vi "VCM_set_values.vi"(4 "Steps":i32=50, 5 "Frequenz":dbl, 6 "A max":dbl, 7 "Amplitude SET":dbl, 8 "mode":u16(ring), 9 "delay time":dbl, 10 "address":string) -> (2 "iter":i32, 3 "Amplitude IST":dbl)   [LabVIEW 2019]
panel:
  out "F-format string":string
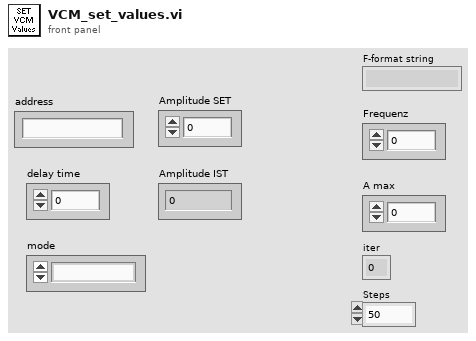
[diagram p1: front panel]
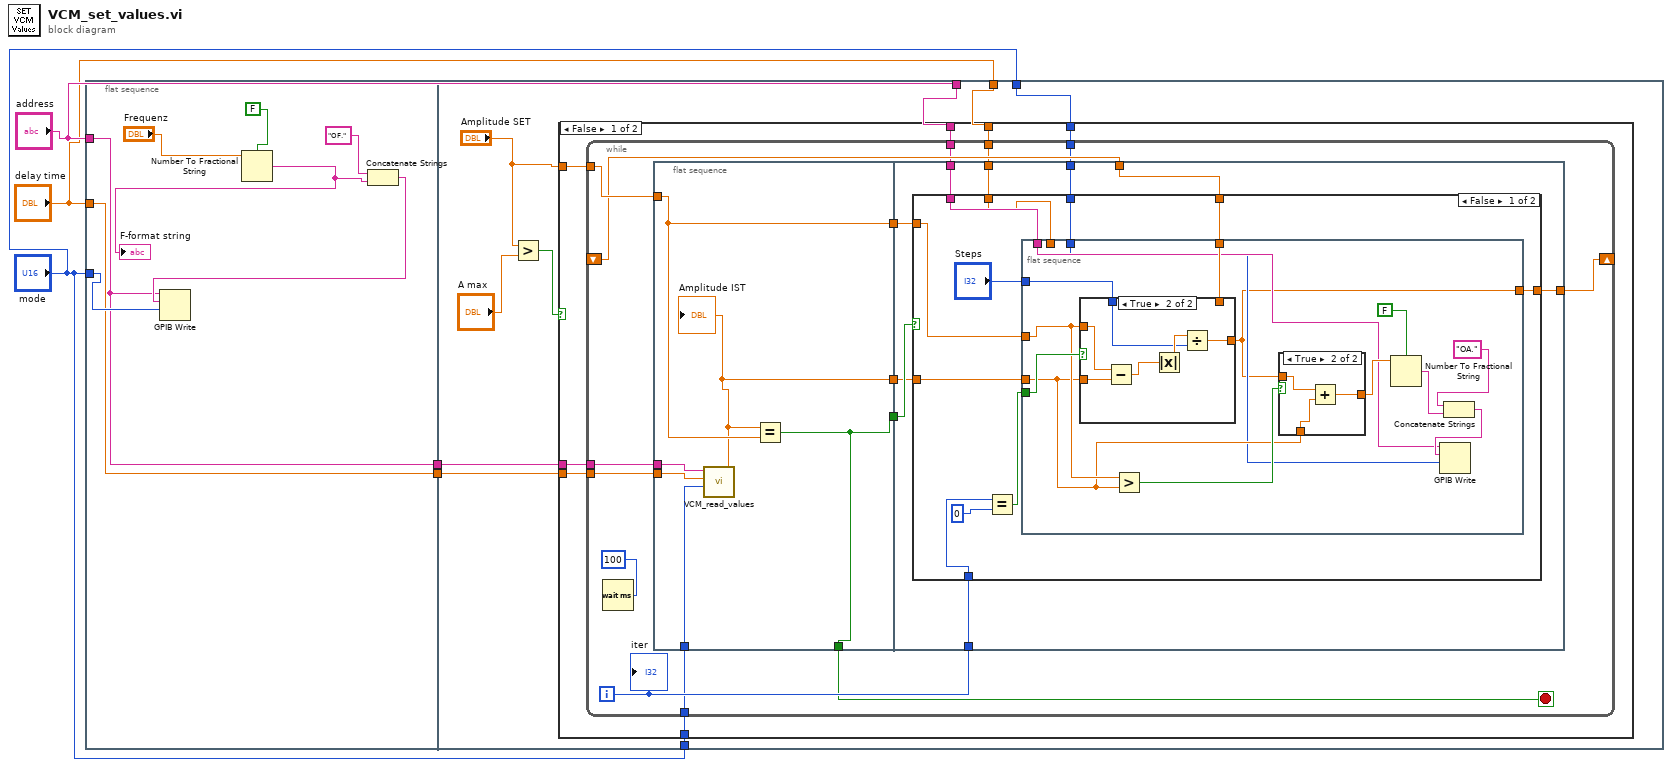
[diagram p0: block diagram]
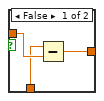
[diagram p2: hidden frame]
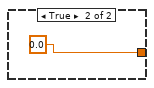
[diagram p4: hidden frame]
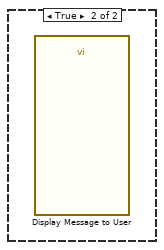
[diagram p5: hidden frame]
diagram:
  n1 = flat-sequence {
    tunnel: "address" -> [w6]
    tunnel: "delay time" -> [w7]
    tunnel: "mode" -> [w10]
    tunnel: [w7] -> w2
    tunnel: [w6] -> w1
    tunnel: "address" -> [w19]
    tunnel: "delay time" -> [w18]
    tunnel: "mode" -> [w17]
    tunnel: "mode" -> [w16]
    tunnel: w2 -> [w15]
    tunnel: w1 -> [w14]
    frame #0 {
      n2 = Number To Fractional String(use system decimal point (T)=FALSE, number="Frequenz") -> (F-format string=w9:string)  [unwired: 2 in]
      "F-format string" <- w9
      n3 = Concatenate Strings("OF.", w9) -> (w8:string)
      n4 = GPIB Write(0:w6, 1:w8, 2:w10) -> ()  [unwired: 2 in, 2 out]
    }
    frame #1 {
      n5 = Greater?(x="Amplitude SET", y="A max") -> (0:w21:bool)
      n6 = case shown="False" w21 {
        tunnel: "Amplitude SET" -> [w29 _]
        tunnel: w19 -> [w28 _]
        tunnel: w18 -> [w27 _]
        tunnel: w17 -> [w26 _]
        tunnel: w16 -> [w25 _]
        tunnel: w15 -> [w24 _]
        tunnel: w14 -> [w23 _]
        frame False {
          n7 = while {
            tunnel: w29 -> [w43]
            shift-right: [w34] -> _
            shift-left: _ -> [w42]
            tunnel: w28 -> [w38]
            tunnel: w27 -> [w37]
            tunnel: w26 -> [w36]
            tunnel: w25 -> [w32]
            tunnel: w24 -> [w31]
            tunnel: w23 -> [w30]
            i -> [w40]
            stop <- w33 stop-if-true
            n8 = Wait (ms)(milliseconds to wait=100) -> ()  [unwired: 1 out]
            n9 = flat-sequence {
              tunnel: w43 -> [w50]
              tunnel: [w49] -> w41
              tunnel: [w50] -> w39
              tunnel: [w45] -> w35
              tunnel: [w49] -> w33
              tunnel: w32 -> [w48]
              tunnel: w31 -> [w47]
              tunnel: w30 -> [w46]
              tunnel: w42 -> [w52]
              tunnel: w41 -> [w59]
              tunnel: w40 -> [w58]
              tunnel: w39 -> [w57]
              tunnel: w38 -> [w56]
              tunnel: w37 -> [w55]
              tunnel: w36 -> [w54]
              tunnel: w35 -> [w53]
              tunnel: [w51] -> w34
              frame #0 {
                n10 = call "VCM_read_values.vi"("mode"=w48, "delay time"=w47, "address"=w46) -> ("Amplitude IST"=w45:dbl)  [unwired: 2 in, 1 out]
                "Amplitude IST" <- w45
                n11 = Equal?(x=w45, y=w50) -> (x = y?=w49:bool)
              }
              frame #1 {
                n12 = case shown="False" w59 {
                  tunnel: w58 -> [w69 _]
                  tunnel: w57 -> [w66 _]
                  tunnel: w56 -> [w65 _]
                  tunnel: w55 -> [w64 _]
                  tunnel: w54 -> [w63 _]
                  tunnel: w53 -> [w62 _]
                  tunnel: w52 -> [w61 _]
                  tunnel: [w60 0.0] -> w51
                  frame False {
                    n13 = Equal?(x=w69, y=0) -> (x = y?=w67:bool)
                    n14 = flat-sequence {
                      tunnel: "Steps" -> [w83]
                      tunnel: w67 -> [w84]
                      tunnel: w66 -> [w81]
                      tunnel: w65 -> [w73]
                      tunnel: w64 -> [_]
                      tunnel: w63 -> [w72]
                      tunnel: w62 -> [w79]
                      tunnel: w61 -> [w82]
                      tunnel: [w71] -> w60
                      frame #0 {
                        n15 = case shown="True" w84 {
                          tunnel: w81 -> [_ w97]
                          tunnel: w79 -> [_ w96]
                          tunnel: w83 -> [_ w93]
                          tunnel: [w91 w92] -> w71
                          tunnel: w82 -> [w91 _]
                          frame False {
                          }
                          frame True {
                            n16 = Subtract(x=w97, y=w96) -> (x-y=w95:dbl)
                            n17 = Absolute Value(x=w95) -> (abs(x)=w94:dbl)
                            n18 = Divide(x=w94, y=w93) -> (x/y=w92:dbl)
                          }
                        }
                        n19 = Greater?(x=w81, y=w79) -> (0:w80:bool)
                        n20 = case shown="True" w80 {
                          tunnel: w71 -> [w87 w90]
                          tunnel: w79 -> [w86 w89]
                          tunnel: [w85 w88] -> w78
                          frame False {
                            n21 = Subtract(x=w86, y=w87) -> (x-y=w85:dbl)
                          }
                          frame True {
                            n22 = Add(x=w90, y=w89) -> (x+y=w88:dbl)
                          }
                        }
                        n23 = Number To Fractional String(use system decimal point (T)=FALSE, number=w78) -> (F-format string=w76:string)  [unwired: 2 in]
                        n24 = Concatenate Strings("OA.", w76) -> (w74:string)
                        n25 = GPIB Write(0:w73, 1:w74, 2:w72) -> ()  [unwired: 2 in, 2 out]
                      }
                    }
                  }
                  frame True {
                  }
                }
              }
            }
            "iter" <- w40
          }
        }
        frame True {
          n26 = call "Display Message to User"() -> ()  [unwired: 10 in, 2 out]
        }
      }
    }
  }
